vi "Forward Data.vi"(8 "error in (no error)":errorcluster, 10 "Data":string, 11 "TCP Read in":refnum<class "TCP Read.lvclass">) -> (0 "error out":errorcluster, 3 "TCP Read out":refnum<class "TCP Read.lvclass">)   [LabVIEW 2017, in "TCP Client.lvlib" / "TCP Read.lvclass"]
doc: "This VI sends the TCP Server \"Incoming Data\" Response directly from the TCP Read Worker to maximise streaming efficiency."
uses:
  TCP Read.lvclass
  TCP Read.lvclass/TCP Read.ctl
  TCP Client/rsp_Incoming Data.ctl
  TCP Client/TCP Client.lvclass
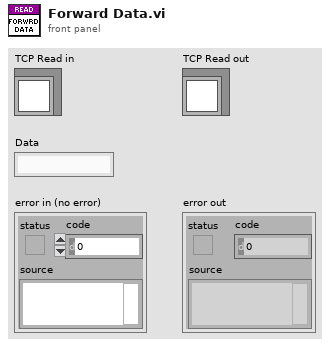
[diagram p1: front panel]
types:
  T1 = typedef "TCP Client.lvlib/TCP Client.lvclass/rsp_Incoming Data.ctl" = cluster{"Data":string}
  T2 = typedef "Workers.lvlib/Case Label.ctl" = string
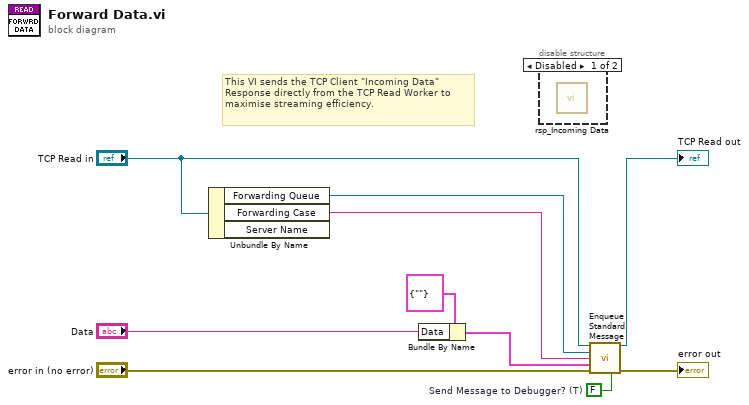
[diagram p0: block diagram]
diagram:
  w10 = FALSE  # Send Message to Debugger? (T)
  # "This VI sends the TCP Client \"Incoming Data\" Response directly from the TCP Read Worker to maximise streaming efficiency."
  n1 = Unbundle By Name("TCP Read in") -> ("Forwarding Queue"=w5:refnum<class "Message Queue.lvclass">, "Forwarding Case"=w4:T2)  [unwired: 1 out]
  n2 = Bundle By Name(cluster=T1 {"Data"=""} ("Data"), "Data"="Data") -> (w3:T1)
  n3 = disable-structure shown="Disabled" {
    frame Disabled {
      n4 = call "rsp_Incoming Data.vi"() -> ()  [unwired: 10 in, 2 out]
    }
    frame Enabled {
    }
  }
  n5 = call-dynamic "Enqueue Standard Message.vi"("Worker"="TCP Read in", "Message Queue"=w5, "Case Label"=w4, "Data"=w3, "error in (no error)"="error in (no error)", "Send Message to Debugger? (T)"=w10) -> ("dup Worker out"=→"TCP Read out":refnum<class "TCP Read.lvclass">, "error out"=→"error out":errorcluster)  [unwired: 8 in]
